vi "mc listbox set active cell (SubVI).vi"(8 "error in (no error)":errorcluster, 9 "row (0)":i32, 10 "column (0)":i32, 11 "multicolumn listbox refnum":refnum<vi>) -> (0 "error out":errorcluster, 3 "multicolumn listbox refnum out":refnum<vi>)   [LabVIEW 2021]
uses:
  <vilib>/Utility/miscctls.llb/LVRowAndColumnTypeDef.ctl
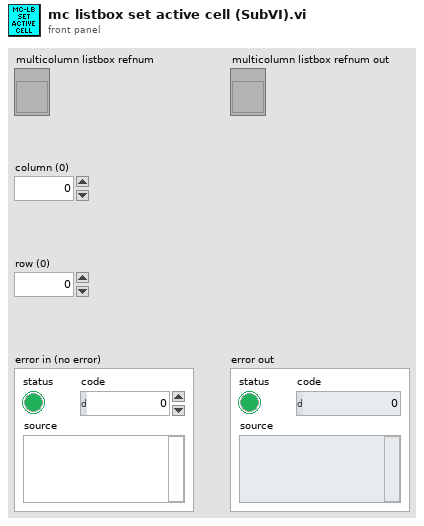
[diagram p1: front panel]
types:
  T1 = typedef "LVRowAndColumnTypeDef.ctl" = cluster{"Row":i32, "Column":i32}
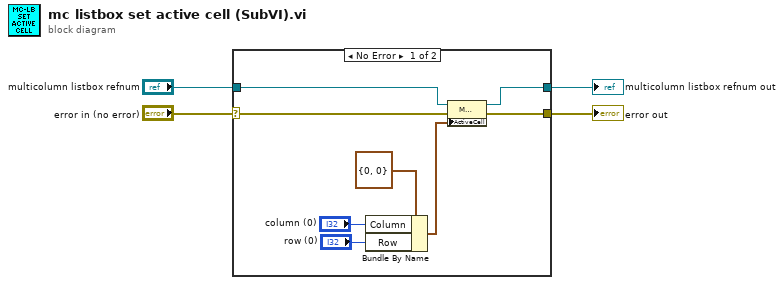
[diagram p0: block diagram]
diagram:
  n1 = case shown="No Error" "error in (no error)" {
    selector: "error in (no error)" -> [w9 w14]
    tunnel: [w12 w13] -> w4
    tunnel: [w11 w14] -> w3
    tunnel: "multicolumn listbox refnum" -> [w10 w13]
    frame No Error {
      n2 = Bundle By Name(cluster=T1 {"Row"=0, "Column"=0} ("Active Cell:Active Cell"), "Column"="column (0)", "Row"="row (0)") -> (w8:T1)
      n3 = property on="Property Node" class="MCListbox (strict)"(reference=w10, error in=w9, "ActiveCell"=w8) -> (reference out=w12:refnum<vi>, error out=w11:errorcluster)
    }
    frame Error {
    }
  }
  "multicolumn listbox refnum out" <- w4
  "error out" <- w3
